vi "Update Fcurve seg bool.vi"(0 "Fcurve Seg":bool, 5 "error in (no error)":errorcluster) -> (19 "error out":errorcluster)   [LabVIEW 2019, in "metadata.lvclass"]
doc: "updates the booleans of the class attribute to know which metadata is available to save"
uses:
  metadata.lvclass
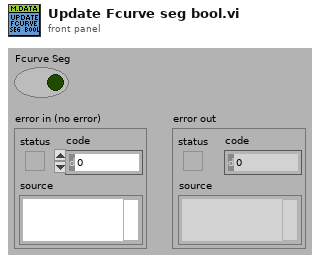
[diagram p1: front panel]
types:
  T1 = typedef "metadata.lvclass/ClassAttributesRef.ctl" = refnum<data-value>
  T2 = typedef "metadata.lvclass/ClassAttributes.ctl" = cluster{"File":bool, "Cantilever":bool, "System control":bool, "XYZ piezos":bool, "Sample info":bool, "Fast fpga param":bool, "Mapping param":bool, "Chirp param":bool, "Fcurve Seg":bool, "Property names":cluster{"File info":string[], "Cantilever calib":string[], "System control":string[], "XYZ piezos":string[], "Sample info":string[], "Fast fpga param":string[], "Mapping param":string[], "Chirp Param":string[], "Fcurve Seg":string[]}}
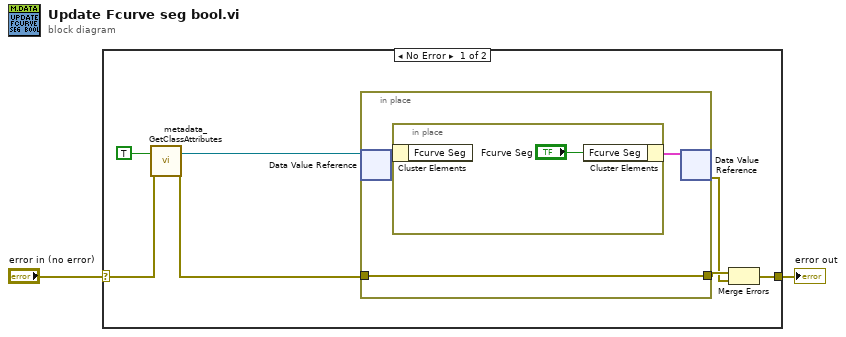
[diagram p0: block diagram]
diagram:
  n1 = case shown="No Error" "error in (no error)" {
    selector: "error in (no error)" -> [w9 w14]
    tunnel: [w6 w14] -> w1
    frame No Error {
      n2 = call "metadata_GetClassAttributes.vi"("return data? (T)"=TRUE ("return data"), "error in (no error)"=w9) -> ("class attributes ref"=w7:T1, "error out"=w8:errorcluster)  [unwired: 14 in, 2 out]
      n3 = in-place {
        in-place-border: w8 -> [w10]
        in-place-border: [w10] -> w4
        n4 = in-place-dvr #1(w7) -> (w11:T2)  [unwired: 1 out]
        n5 = in-place {
          n6 = in-place-cluster #2(w11) -> ()  [unwired: 1 out]
          n7 = in-place-cluster #2("Fcurve Seg"="Fcurve Seg") -> (w12:T2)
        }
        n8 = in-place-dvr #1(w12) -> (w3:errorcluster)  [unwired: 1 out]
      }
      n9 = Merge Errors(w4, w3) -> (w6:errorcluster)
    }
    frame Error {
    }
  }
  "error out" <- w1
